vi "Autonomous Independent.vi"() -> ()   [LabVIEW 2014]
doc: "This VI is called when autonomous begins, and will automatically be terminated when autonomous ends. You can carry out timed or sensor driven robot movement independently without needing to return to the caller."
uses:
  <vilib>/Rock Robotics/WPI/Solenoid/WPI_SolenoidValue.ctl
  <vilib>/Rock Robotics/WPI/Solenoid/WPI_SolenoidSetEnum.vi
  <vilib>/Rock Robotics/WPI/RobotDrive/WPI_RobotDriveGetSetRefNum.vi
  <vilib>/Rock Robotics/WPI/RobotDrive/WPI_RobotDriveArcadeDrive_Standard(NoSaturation).vi
panel:
  out "Out":dbl
  # "Be sure to right-click and choose Data Operations>>Make Current Value default if you want to save the array values with the VI"
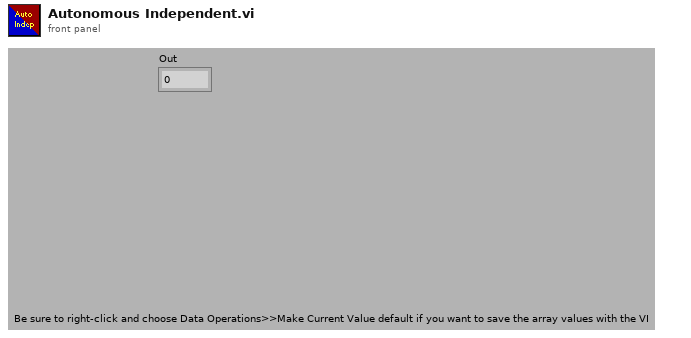
[diagram p1: front panel]
types:
  T1 = typedef "WPI_DigitalInputDevRef.ctl" = cluster{"DevStatus":errorcluster, "DIO Channel":T2, "Controller":T3}
  T2 = typedef "FPGA_DIOChannel.ctl" = enum8{"DIO 0", "DIO 1", "DIO 2", "DIO 3", "DIO 4", "DIO 5", "DIO 6", "DIO 7", "DIO 8", "DIO 9", "DIO MXP 0", "DIO MXP 1", "DIO MXP 2", "DIO MXP 3", "DIO MXP 4", "DIO MXP 5", "DIO MXP 6", "DIO MXP 7", "DIO MXP 8", "DIO MXP 9", "DIO MXP 10", "DIO MXP 11", "DIO MXP 12", "DIO MXP 13", "DIO MXP 14", "DIO MXP 15", "Invalid"}
  T3 = typedef "FPGA_TypedefDigitalModule.ctl" = enum16{"Controller 1"}
  T4 = typedef "WPI_SolenoidValue.ctl" = enum16{"Off", "On", "Forward", "Reverse"}
  T5 = typedef "WPI_SolenoidDevRef.ctl" = cluster{"DevStatus":errorcluster, "Pneumatics Control Module":u8, "Forward Solenoid Channel":T6, "Reverse Solenoid Channel":T6}
  T6 = typedef "WPI_SolenoidChannel.ctl" = enum8{"Solenoid 0", "Solenoid 1", "Solenoid 2", "Solenoid 3", "Solenoid 4", "Solenoid 5", "Solenoid 6", "Solenoid 7", "Invalid"}
  T7 = typedef "WPI_EncoderDevRef.ctl" = cluster{"DevStatus":errorcluster, "EncoderIndex":T8, "CounterIndex":T9, "DistancePerCount":dbl, "Decoding Type":T10}
  T8 = typedef "FPGA_EncoderIdx.ctl" = enum8{"Enc 0", "Enc 1", "Enc 2", "Enc 3", "Enc 4", "Enc 5", "Enc 6", "Enc 7", "Invalid"}
  T9 = typedef "FPGA_CounterCtrSystemIndex.ctl" = enum8{"Ctr 0", "Ctr 1", "Ctr 2", "Ctr 3", "Ctr 4", "Ctr 5", "Ctr 6", "Ctr 7", "Invalid"}
  T10 = typedef "WPI_EncoderType.ctl" = enum16{"1x", "2x", "4x"}
  T11 = typedef "WPI_RobotDriveDevRef.ctl" = cluster{"DevStatus":errorcluster, "Motors[]":T12[], "Square Inputs":bool, "Max Output":dbl}
  T12 = typedef "WPI_MotorControlDeviceRef.ctl" = cluster{"DeviceStatus":errorcluster, "Type":T13, "PWM":cluster{"Controller":T3, "PWM Channel":T14, "DeadBand":T15}, "CAN":cluster{"Device Number":u8, "Control Mode":T16, "Semaphore":T17, "Max Vout":dbl, "TalonSRX Control Mode":T18}, "Invert":bool, "TransformRef":T19, "InvTransformRef":T19}
  T13 = typedef "WPI_MotorControlType.ctl" = enum16{"PWM", "CAN", "CANTalonSRX"}
  T14 = typedef "FPGA_DIOPWMChannel.ctl" = enum8{"PWM 0", "PWM 1", "PWM 2", "PWM 3", "PWM 4", "PWM 5", "PWM 6", "PWM 7", "PWM 8", "PWM 9", "PWM MXP 0", "PWM MXP 1", "PWM MXP 2", "PWM MXP 3", "PWM MXP 4", "PWM MXP 5", "PWM MXP 6", "PWM MXP 7", "PWM MXP 8", "PWM MXP 9", "Invalid"}
  T15 = typedef "WPI_PWMDeadband.ctl" = cluster{"Name":string, "maxPositivePwm":i32, "minPositivePwm":i32, "centerPwm":i32, "maxNegativePwm":i32, "minNegativePwm":i32, "angularRange":u16}
  T16 = typedef "WPI_CANJaguar_ControlMode.ctl" = enum8{"Percent VBus", "Current", "Speed", "Position", "Voltage"}
  T17 = typedef "Semaphore RefNum" = refnum<k1>
  T18 = typedef "WPI_CANTalonSRX_APIControlMode.ctl" = enum8{"Percent VBus", "Speed", "Position", "Slave", "Unchanged / Invalid"}
  T19 = typedef "WPI_PWMTransform_ConPane.ctl" = refnum<vi>
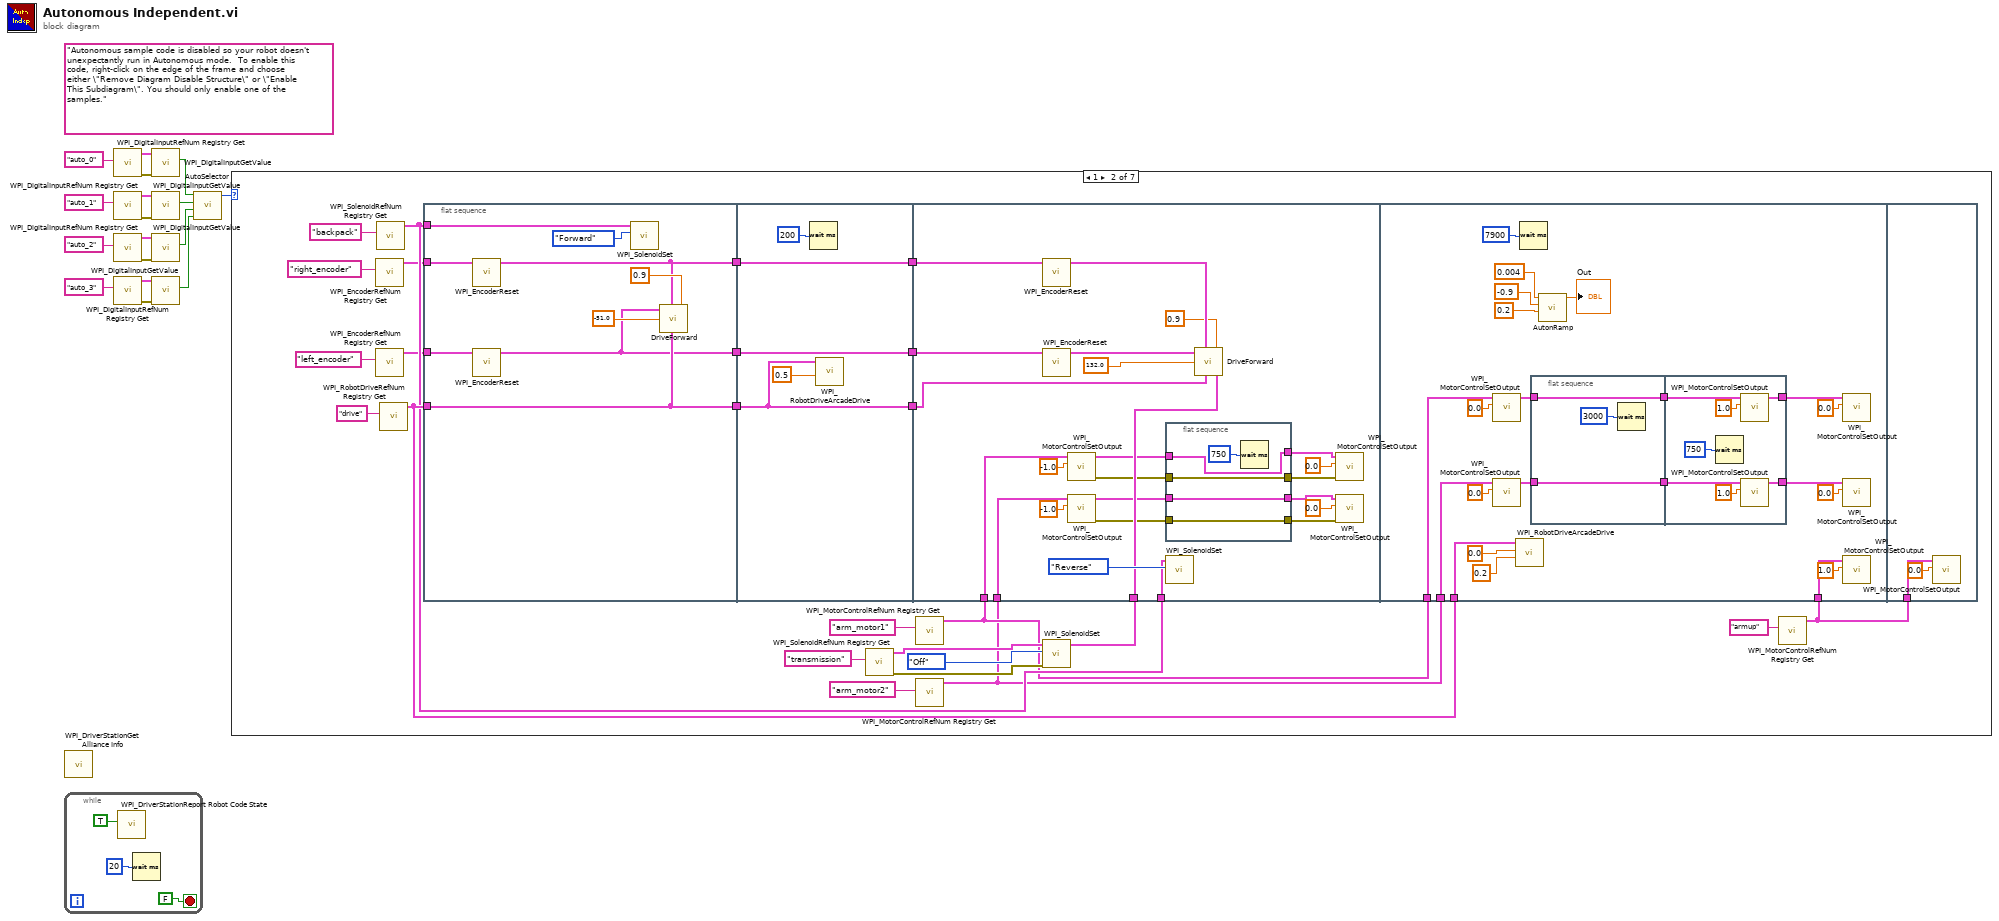
[diagram p0: block diagram]
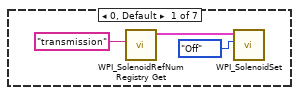
[diagram p2: hidden frame]
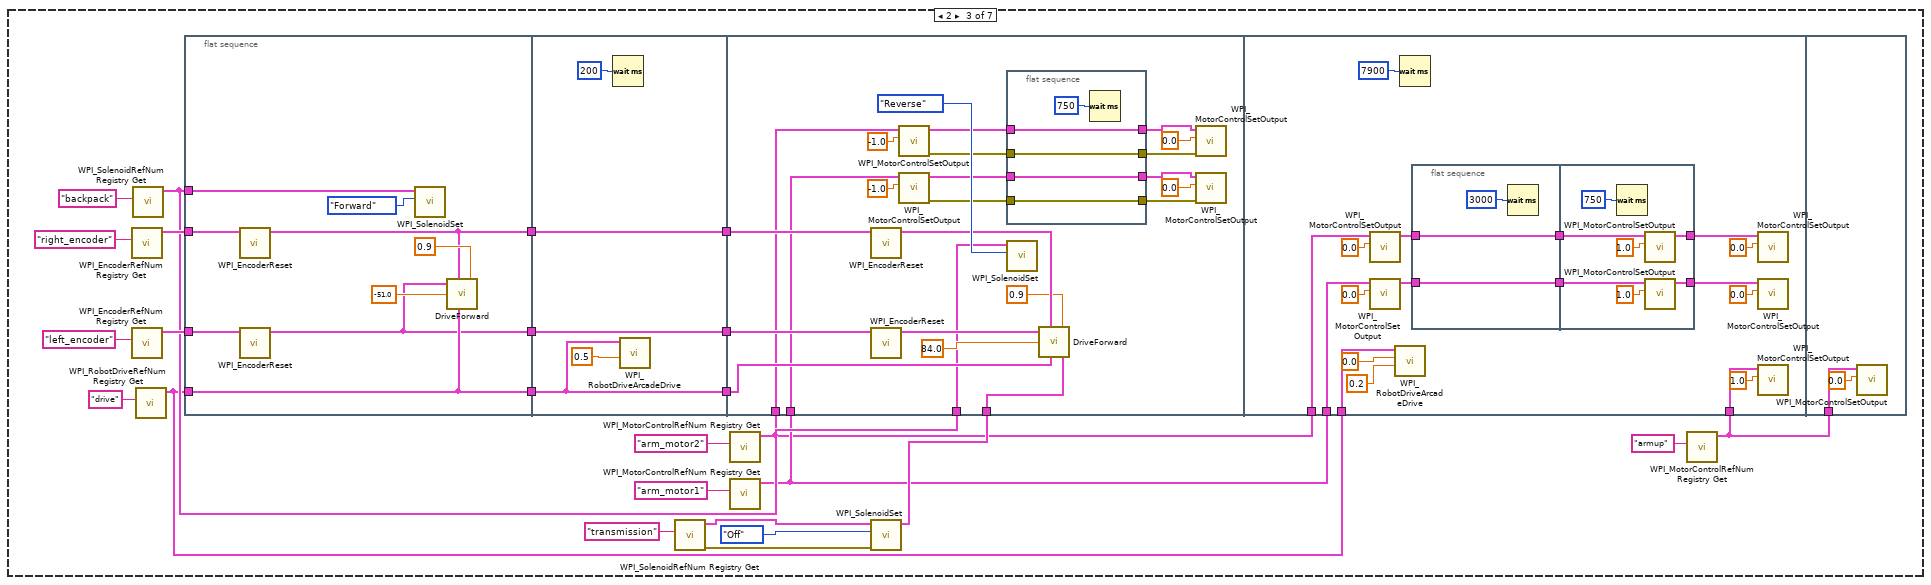
[diagram p3: hidden frame]
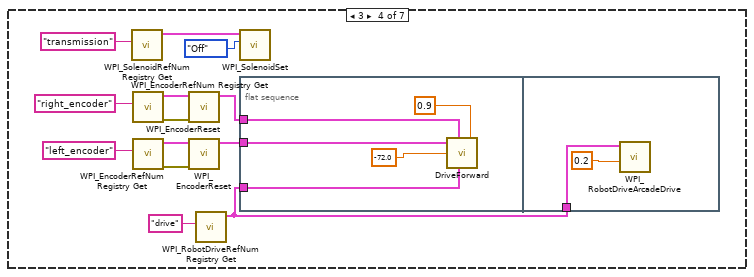
[diagram p4: hidden frame]
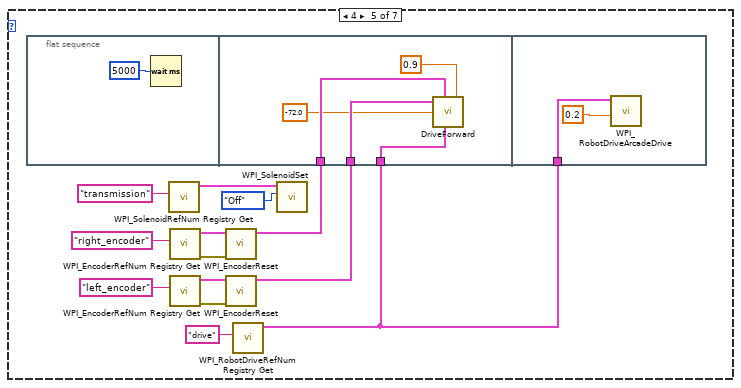
[diagram p5: hidden frame]
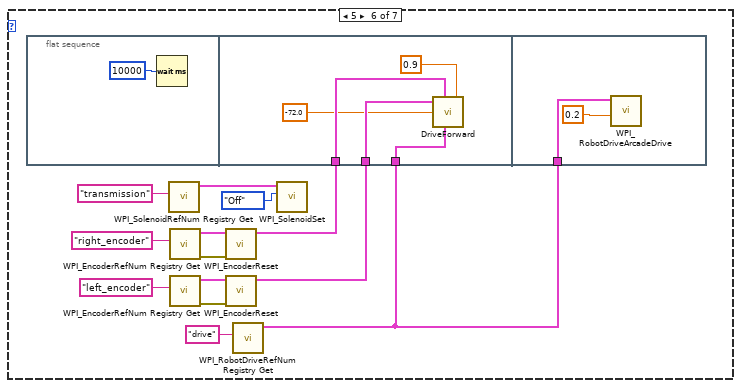
[diagram p6: hidden frame]
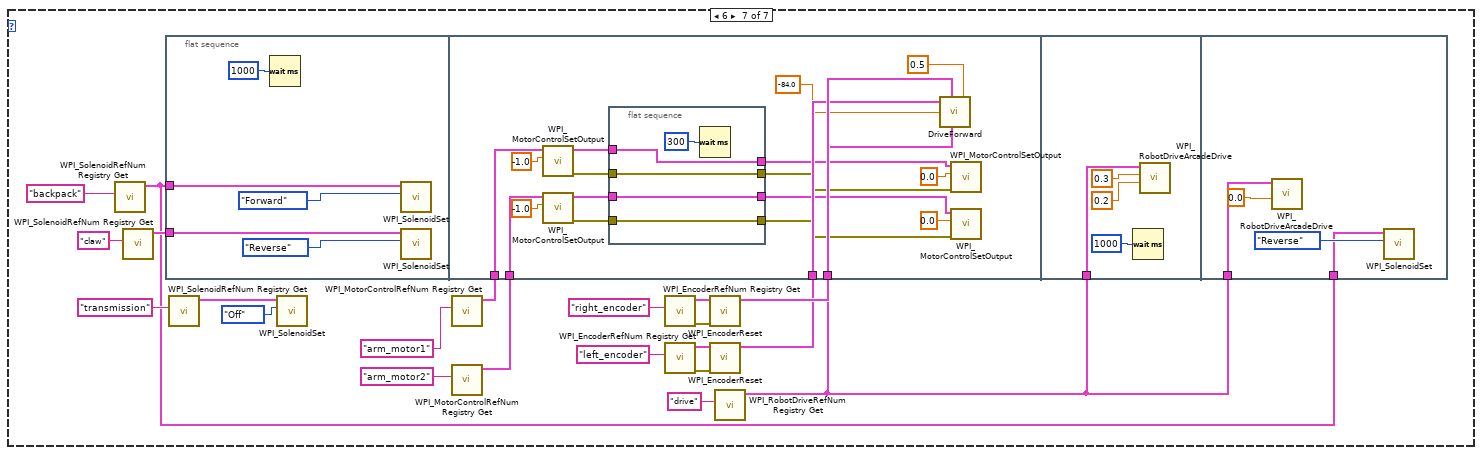
[diagram p7: hidden frame]
diagram:
  (unwired) "Autonomous sample code is disabled so your robot doesn't unexpectantly run in Autonomous mode.  To enable this code, right-click on the edge of the frame and choose either \"Remove Diagram Disable Structure\" or \"Enable This Subdiagram\". You should only enable one of the samples."
  n1 = call <vilib>:"WPI_DriverStationGet Alliance Info.vi"() -> ()  [unwired: 12 out]
  n2 = while {
    stop <- FALSE stop-if-true
    n3 = call <vilib>:"WPI_DriverStationReport Robot Code State.vi"("Autonomous"=TRUE) -> ()  [unwired: 10 in, 1 out]
    n4 = Wait (ms)(milliseconds to wait=u32 20) -> ()  [unwired: 1 out]
  }
  n5 = call <vilib>:"WPI_DigitalInputRefNum Registry Get.vi"("refnum name"="auto_0") -> ("error out"=w16:errorcluster, "DigitalInputDevRef"=w15:T1)  [unwired: 9 in]
  n6 = call <vilib>:"WPI_DigitalInputRefNum Registry Get.vi"("refnum name"="auto_1") -> ("error out"=w13:errorcluster, "DigitalInputDevRef"=w14:T1)  [unwired: 9 in]
  n7 = call <vilib>:"WPI_DigitalInputRefNum Registry Get.vi"("refnum name"="auto_2") -> ("error out"=w11:errorcluster, "DigitalInputDevRef"=w12:T1)  [unwired: 9 in]
  n8 = call <vilib>:"WPI_DigitalInputRefNum Registry Get.vi"("refnum name"="auto_3") -> ("error out"=w9:errorcluster, "DigitalInputDevRef"=w10:T1)  [unwired: 9 in]
  n9 = call <vilib>:"WPI_DigitalInputGetValue.vi"("error in (no error)"=w16, "DigitalInputDevRef"=w15) -> ("Value"=w5:bool)  [unwired: 7 in, 2 out]
  n10 = call <vilib>:"WPI_DigitalInputGetValue.vi"("error in (no error)"=w13, "DigitalInputDevRef"=w14) -> ("Value"=w6:bool)  [unwired: 7 in, 2 out]
  n11 = call <vilib>:"WPI_DigitalInputGetValue.vi"("error in (no error)"=w11, "DigitalInputDevRef"=w12) -> ("Value"=w7:bool)  [unwired: 7 in, 2 out]
  n12 = call <vilib>:"WPI_DigitalInputGetValue.vi"("error in (no error)"=w9, "DigitalInputDevRef"=w10) -> ("Value"=w8:bool)  [unwired: 7 in, 2 out]
  n13 = call "AutoSelector.vi"("3"=w8, "2"=w7, "1"=w6, "0"=w5) -> ("Auto"=w17:i32)  [unwired: 7 in]
  n14 = case shown="1" w17 {
    frame 0, Default {
      n15 = call <vilib>:"WPI_SolenoidRefNum Registry Get.vi"("refnum name"="transmission") -> ("SolenoidDevRef"=w21:T5)  [unwired: 9 in, 1 out]
      n16 = call-poly <vilib>:"WPI_SolenoidSet.vi"("Value"=WPI_SolenoidValue."Off", "SolenoidDevRef"=w21) -> ()  [unwired: 8 in, 2 out]
    }
    frame 1 {
      n17 = call <vilib>:"WPI_EncoderRefNum Registry Get.vi"("refnum name"="right_encoder") -> ("EncoderDevRef"=w34:T7)  [unwired: 9 in, 1 out]
      n18 = call <vilib>:"WPI_EncoderRefNum Registry Get.vi"("refnum name"="left_encoder") -> ("EncoderDevRef"=w35:T7)  [unwired: 9 in, 1 out]
      n19 = call <vilib>:"WPI_SolenoidRefNum Registry Get.vi"("refnum name"="backpack") -> ("SolenoidDevRef"=w36:T5)  [unwired: 9 in, 1 out]
      n20 = call <vilib>:"WPI_RobotDriveRefNum Registry Get.vi"("refnum name"="drive") -> ("RobotDriveDevRef"=w42:T11)  [unwired: 9 in, 1 out]
      n21 = flat-sequence {
        tunnel: w42 -> [w53]
        tunnel: w34 -> [w49]
        tunnel: w35 -> [w50]
        tunnel: w36 -> [w57]
        tunnel: [w53] -> w48
        tunnel: [w52] -> w47
        tunnel: [w51] -> w46
        tunnel: w48 -> [w59]
        tunnel: [w59] -> w45
        tunnel: w47 -> [w62]
        tunnel: [w62] -> w44
        tunnel: w46 -> [w61]
        tunnel: [w61] -> w43
        tunnel: w45 -> [w81]
        tunnel: w44 -> [w80]
        tunnel: w43 -> [w79]
        tunnel: w36 -> [w78]
        tunnel: w37 -> [w77]
        tunnel: w25 -> [w64]
        tunnel: w24 -> [w63]
        tunnel: w41 -> [w111]
        tunnel: w42 -> [w108]
        tunnel: w25 -> [w93]
        tunnel: w24 -> [w92]
        tunnel: w41 -> [w124]
        frame #0 {
          n22 = call <vilib>:"WPI_EncoderReset.vi"("EncoderDevRef"=w49) -> ("EncoderDevRef"=w51:T7)  [unwired: 9 in, 1 out]
          n23 = call <vilib>:"WPI_EncoderReset.vi"("EncoderDevRef"=w50) -> ("EncoderDevRef"=w52:T7)  [unwired: 9 in, 1 out]
          n24 = call-poly <vilib>:"WPI_SolenoidSet.vi"("Value"=WPI_SolenoidValue."Forward", "SolenoidDevRef"=w57) -> ()  [unwired: 8 in, 2 out]
          n25 = call "DriveForward.vi"("LeftEncoder"=w52, "RightEncoder"=w51, "Inches to Travel"=-51.0, "Drive"=w53, "Max"=0.9) -> ()  [unwired: 2 in]
        }
        frame #1 {
          n26 = Wait (ms)(milliseconds to wait=u32 200) -> ()  [unwired: 1 out]
          n27 = call-poly <vilib>:"WPI_RobotDriveArcadeDrive.vi"("Y axis value"=0.5, "RobotDriveDevRef"=w59) -> ()  [unwired: 7 in, 3 out]
        }
        frame #2 {
          n28 = call <vilib>:"WPI_EncoderReset.vi"("EncoderDevRef"=w79) -> ("EncoderDevRef"=w84:T7)  [unwired: 9 in, 1 out]
          n29 = call <vilib>:"WPI_EncoderReset.vi"("EncoderDevRef"=w80) -> ("EncoderDevRef"=w85:T7)  [unwired: 9 in, 1 out]
          n30 = call <vilib>:"WPI_MotorControlSetOutput.vi"("Output"=-1.0, "MotorControlDevRef"=w64) -> ("error out"=w68:errorcluster, "MotorControlDevRef"=w76:T12)  [unwired: 7 in, 1 out]
          n31 = call <vilib>:"WPI_MotorControlSetOutput.vi"("Output"=-1.0, "MotorControlDevRef"=w63) -> ("error out"=w67:errorcluster, "MotorControlDevRef"=w73:T12)  [unwired: 7 in, 1 out]
          n32 = flat-sequence {
            tunnel: w67 -> [w90]
            tunnel: w68 -> [w91]
            tunnel: [w91] -> w69
            tunnel: [w90] -> w70
            tunnel: w73 -> [w88]
            tunnel: [w88] -> w74
            tunnel: [w87] -> w75
            tunnel: w76 -> [w87]
            frame #0 {
              n33 = Wait (ms)(milliseconds to wait=u32 750) -> ()  [unwired: 1 out]
            }
          }
          n34 = call-poly <vilib>:"WPI_SolenoidSet.vi"("Value"=WPI_SolenoidValue."Reverse", "SolenoidDevRef"=w78) -> ()  [unwired: 8 in, 2 out]
          n35 = call "DriveForward.vi"("LeftEncoder"=w85, "RightEncoder"=w84, "Inches to Travel"=132.0, "Drive"=w81, "Max"=0.9, "Transmission"=w77) -> ()  [unwired: 1 in]
          n36 = call <vilib>:"WPI_MotorControlSetOutput.vi"("error in (no error)"=w69, "Output"=0.0, "MotorControlDevRef"=w75) -> ()  [unwired: 6 in, 3 out]
          n37 = call <vilib>:"WPI_MotorControlSetOutput.vi"("error in (no error)"=w70, "Output"=0.0, "MotorControlDevRef"=w74) -> ()  [unwired: 6 in, 3 out]
        }
        frame #3 {
          n38 = call <vilib>:"WPI_MotorControlSetOutput.vi"("Output"=0.0, "MotorControlDevRef"=w93) -> ("MotorControlDevRef"=w98:T12)  [unwired: 7 in, 2 out]
          n39 = call <vilib>:"WPI_MotorControlSetOutput.vi"("Output"=0.0, "MotorControlDevRef"=w92) -> ("MotorControlDevRef"=w99:T12)  [unwired: 7 in, 2 out]
          n40 = call-poly <vilib>:"WPI_RobotDriveArcadeDrive.vi"("Y axis value"=0.2, "X axis value"=0.0 ("Y axis value"), "RobotDriveDevRef"=w108) -> ()  [unwired: 6 in, 3 out]
          n41 = Wait (ms)(milliseconds to wait=u32 7900) -> ()  [unwired: 1 out]
          n42 = flat-sequence {
            tunnel: w99 -> [w115]
            tunnel: w98 -> [w114]
            tunnel: [w115] -> w103
            tunnel: [w114] -> w102
            tunnel: w103 -> [w120]
            tunnel: w102 -> [w119]
            tunnel: [w117] -> w96
            tunnel: [w118] -> w97
            frame #0 {
              n43 = Wait (ms)(milliseconds to wait=u32 3000) -> ()  [unwired: 1 out]
            }
            frame #1 {
              n44 = Wait (ms)(milliseconds to wait=u32 750) -> ()  [unwired: 1 out]
              n45 = call <vilib>:"WPI_MotorControlSetOutput.vi"("Output"=1.0, "MotorControlDevRef"=w119) -> ("MotorControlDevRef"=w117:T12)  [unwired: 7 in, 2 out]
              n46 = call <vilib>:"WPI_MotorControlSetOutput.vi"("Output"=1.0, "MotorControlDevRef"=w120) -> ("MotorControlDevRef"=w118:T12)  [unwired: 7 in, 2 out]
            }
          }
          n47 = call "AutonRamp.vi"("Target"=0.2, "Start"=-0.9, "Rate"=0.004) -> ("Out"=→"Out":dbl)  [unwired: 8 in]
          n48 = call <vilib>:"WPI_MotorControlSetOutput.vi"("Output"=0.0, "MotorControlDevRef"=w96) -> ()  [unwired: 7 in, 3 out]
          n49 = call <vilib>:"WPI_MotorControlSetOutput.vi"("Output"=0.0, "MotorControlDevRef"=w97) -> ()  [unwired: 7 in, 3 out]
          n50 = call <vilib>:"WPI_MotorControlSetOutput.vi"("Output"=1.0, "MotorControlDevRef"=w111) -> ()  [unwired: 7 in, 3 out]
        }
        frame #4 {
          n51 = call <vilib>:"WPI_MotorControlSetOutput.vi"("Output"=0.0, "MotorControlDevRef"=w124) -> ()  [unwired: 7 in, 3 out]
        }
      }
      n52 = call <vilib>:"WPI_SolenoidRefNum Registry Get.vi"("refnum name"="transmission") -> ("error out"=w29:errorcluster, "SolenoidDevRef"=w30:T5)  [unwired: 9 in]
      n53 = call <vilib>:"WPI_MotorControlRefNum Registry Get.vi"("refnum name"="arm_motor1") -> ("MotorControlDevRef"=w25:T12)  [unwired: 9 in, 1 out]
      n54 = call <vilib>:"WPI_MotorControlRefNum Registry Get.vi"("refnum name"="arm_motor2") -> ("MotorControlDevRef"=w24:T12)  [unwired: 9 in, 1 out]
      n55 = call-poly <vilib>:"WPI_SolenoidSet.vi"("error in (no error)"=w29, "Value"=WPI_SolenoidValue."Off", "SolenoidDevRef"=w30) -> ("SolenoidDevRef"=w37:T5)  [unwired: 7 in, 1 out]
      n56 = call <vilib>:"WPI_MotorControlRefNum Registry Get.vi"("refnum name"="armup") -> ("MotorControlDevRef"=w41:T12)  [unwired: 9 in, 1 out]
    }
    frame 2 {
      n57 = call <vilib>:"WPI_EncoderRefNum Registry Get.vi"("refnum name"="right_encoder") -> ("EncoderDevRef"=w136:T7)  [unwired: 9 in, 1 out]
      n58 = call <vilib>:"WPI_EncoderRefNum Registry Get.vi"("refnum name"="left_encoder") -> ("EncoderDevRef"=w135:T7)  [unwired: 9 in, 1 out]
      n59 = call <vilib>:"WPI_SolenoidRefNum Registry Get.vi"("refnum name"="backpack") -> ("SolenoidDevRef"=w134:T5)  [unwired: 9 in, 1 out]
      n60 = call <vilib>:"WPI_RobotDriveRefNum Registry Get.vi"("refnum name"="drive") -> ("RobotDriveDevRef"=w128:T11)  [unwired: 9 in, 1 out]
      n61 = flat-sequence {
        tunnel: w128 -> [w155]
        tunnel: w136 -> [w151]
        tunnel: w135 -> [w152]
        tunnel: w134 -> [w159]
        tunnel: [w155] -> w150
        tunnel: [w154] -> w149
        tunnel: [w153] -> w148
        tunnel: w150 -> [w161]
        tunnel: [w161] -> w147
        tunnel: w149 -> [w164]
        tunnel: [w164] -> w146
        tunnel: w148 -> [w163]
        tunnel: [w163] -> w145
        tunnel: w147 -> [w183]
        tunnel: w146 -> [w182]
        tunnel: w145 -> [w181]
        tunnel: w134 -> [w180]
        tunnel: w133 -> [w179]
        tunnel: w127 -> [w166]
        tunnel: w126 -> [w165]
        tunnel: w129 -> [w209]
        tunnel: w128 -> [w206]
        tunnel: w127 -> [w203]
        tunnel: w126 -> [w202]
        tunnel: w129 -> [w222]
        frame #0 {
          n62 = call <vilib>:"WPI_EncoderReset.vi"("EncoderDevRef"=w151) -> ("EncoderDevRef"=w153:T7)  [unwired: 9 in, 1 out]
          n63 = call <vilib>:"WPI_EncoderReset.vi"("EncoderDevRef"=w152) -> ("EncoderDevRef"=w154:T7)  [unwired: 9 in, 1 out]
          n64 = call-poly <vilib>:"WPI_SolenoidSet.vi"("Value"=WPI_SolenoidValue."Forward", "SolenoidDevRef"=w159) -> ()  [unwired: 8 in, 2 out]
          n65 = call "DriveForward.vi"("LeftEncoder"=w154, "RightEncoder"=w153, "Inches to Travel"=-51.0, "Drive"=w155, "Max"=0.9) -> ()  [unwired: 2 in]
        }
        frame #1 {
          n66 = Wait (ms)(milliseconds to wait=u32 200) -> ()  [unwired: 1 out]
          n67 = call-poly <vilib>:"WPI_RobotDriveArcadeDrive.vi"("Y axis value"=0.5, "RobotDriveDevRef"=w161) -> ()  [unwired: 7 in, 3 out]
        }
        frame #2 {
          n68 = call <vilib>:"WPI_EncoderReset.vi"("EncoderDevRef"=w181) -> ("EncoderDevRef"=w186:T7)  [unwired: 9 in, 1 out]
          n69 = call <vilib>:"WPI_EncoderReset.vi"("EncoderDevRef"=w182) -> ("EncoderDevRef"=w187:T7)  [unwired: 9 in, 1 out]
          n70 = call <vilib>:"WPI_MotorControlSetOutput.vi"("Output"=-1.0, "MotorControlDevRef"=w165) -> ("error out"=w169:errorcluster, "MotorControlDevRef"=w175:T12)  [unwired: 7 in, 1 out]
          n71 = call <vilib>:"WPI_MotorControlSetOutput.vi"("Output"=-1.0, "MotorControlDevRef"=w166) -> ("error out"=w170:errorcluster, "MotorControlDevRef"=w178:T12)  [unwired: 7 in, 1 out]
          n72 = flat-sequence {
            tunnel: w169 -> [w192]
            tunnel: w170 -> [w193]
            tunnel: [w193] -> w171
            tunnel: [w192] -> w172
            tunnel: w175 -> [w190]
            tunnel: [w190] -> w176
            tunnel: [w189] -> w177
            tunnel: w178 -> [w189]
            frame #0 {
              n73 = Wait (ms)(milliseconds to wait=u32 750) -> ()  [unwired: 1 out]
            }
          }
          n74 = call-poly <vilib>:"WPI_SolenoidSet.vi"("Value"=WPI_SolenoidValue."Reverse", "SolenoidDevRef"=w180) -> ()  [unwired: 8 in, 2 out]
          n75 = call "DriveForward.vi"("LeftEncoder"=w187, "RightEncoder"=w186, "Inches to Travel"=84.0, "Drive"=w183, "Max"=0.9, "Transmission"=w179) -> ()  [unwired: 1 in]
          n76 = call <vilib>:"WPI_MotorControlSetOutput.vi"("error in (no error)"=w172, "Output"=0.0, "MotorControlDevRef"=w176) -> ()  [unwired: 6 in, 3 out]
          n77 = call <vilib>:"WPI_MotorControlSetOutput.vi"("error in (no error)"=w171, "Output"=0.0, "MotorControlDevRef"=w177) -> ()  [unwired: 6 in, 3 out]
        }
        frame #3 {
          n78 = call <vilib>:"WPI_MotorControlSetOutput.vi"("Output"=0.0, "MotorControlDevRef"=w202) -> ("MotorControlDevRef"=w200:T12)  [unwired: 7 in, 2 out]
          n79 = call <vilib>:"WPI_MotorControlSetOutput.vi"("Output"=0.0, "MotorControlDevRef"=w203) -> ("MotorControlDevRef"=w201:T12)  [unwired: 7 in, 2 out]
          n80 = call-poly <vilib>:"WPI_RobotDriveArcadeDrive.vi"("Y axis value"=0.2, "X axis value"=0.0 ("Y axis value"), "RobotDriveDevRef"=w206) -> ()  [unwired: 6 in, 3 out]
          n81 = Wait (ms)(milliseconds to wait=u32 7900) -> ()  [unwired: 1 out]
          n82 = flat-sequence {
            tunnel: w201 -> [w213]
            tunnel: w200 -> [w212]
            tunnel: [w213] -> w199
            tunnel: [w212] -> w198
            tunnel: w199 -> [w218]
            tunnel: w198 -> [w217]
            tunnel: [w215] -> w196
            tunnel: [w216] -> w197
            frame #0 {
              n83 = Wait (ms)(milliseconds to wait=u32 3000) -> ()  [unwired: 1 out]
            }
            frame #1 {
              n84 = Wait (ms)(milliseconds to wait=u32 750) -> ()  [unwired: 1 out]
              n85 = call <vilib>:"WPI_MotorControlSetOutput.vi"("Output"=1.0, "MotorControlDevRef"=w217) -> ("MotorControlDevRef"=w215:T12)  [unwired: 7 in, 2 out]
              n86 = call <vilib>:"WPI_MotorControlSetOutput.vi"("Output"=1.0, "MotorControlDevRef"=w218) -> ("MotorControlDevRef"=w216:T12)  [unwired: 7 in, 2 out]
            }
          }
          n87 = call <vilib>:"WPI_MotorControlSetOutput.vi"("Output"=0.0, "MotorControlDevRef"=w196) -> ()  [unwired: 7 in, 3 out]
          n88 = call <vilib>:"WPI_MotorControlSetOutput.vi"("Output"=0.0, "MotorControlDevRef"=w197) -> ()  [unwired: 7 in, 3 out]
          n89 = call <vilib>:"WPI_MotorControlSetOutput.vi"("Output"=1.0, "MotorControlDevRef"=w209) -> ()  [unwired: 7 in, 3 out]
        }
        frame #4 {
          n90 = call <vilib>:"WPI_MotorControlSetOutput.vi"("Output"=0.0, "MotorControlDevRef"=w222) -> ()  [unwired: 7 in, 3 out]
        }
      }
      n91 = call <vilib>:"WPI_SolenoidRefNum Registry Get.vi"("refnum name"="transmission") -> ("error out"=w141:errorcluster, "SolenoidDevRef"=w140:T5)  [unwired: 9 in]
      n92 = call <vilib>:"WPI_MotorControlRefNum Registry Get.vi"("refnum name"="arm_motor2") -> ("MotorControlDevRef"=w126:T12)  [unwired: 9 in, 1 out]
      n93 = call <vilib>:"WPI_MotorControlRefNum Registry Get.vi"("refnum name"="arm_motor1") -> ("MotorControlDevRef"=w127:T12)  [unwired: 9 in, 1 out]
      n94 = call-poly <vilib>:"WPI_SolenoidSet.vi"("error in (no error)"=w141, "Value"=WPI_SolenoidValue."Off", "SolenoidDevRef"=w140) -> ("SolenoidDevRef"=w133:T5)  [unwired: 7 in, 1 out]
      n95 = call <vilib>:"WPI_MotorControlRefNum Registry Get.vi"("refnum name"="armup") -> ("MotorControlDevRef"=w129:T12)  [unwired: 9 in, 1 out]
    }
    frame 3 {
      n96 = call <vilib>:"WPI_SolenoidRefNum Registry Get.vi"("refnum name"="transmission") -> ("SolenoidDevRef"=w224:T5)  [unwired: 9 in, 1 out]
      n97 = call <vilib>:"WPI_EncoderRefNum Registry Get.vi"("refnum name"="right_encoder") -> ("error out"=w229:errorcluster, "EncoderDevRef"=w232:T7)  [unwired: 9 in]
      n98 = call <vilib>:"WPI_EncoderRefNum Registry Get.vi"("refnum name"="left_encoder") -> ("error out"=w230:errorcluster, "EncoderDevRef"=w231:T7)  [unwired: 9 in]
      n99 = call <vilib>:"WPI_EncoderReset.vi"("error in (no error)"=w229, "EncoderDevRef"=w232) -> ("EncoderDevRef"=w228:T7)  [unwired: 8 in, 1 out]
      n100 = call <vilib>:"WPI_EncoderReset.vi"("error in (no error)"=w230, "EncoderDevRef"=w231) -> ("EncoderDevRef"=w227:T7)  [unwired: 8 in, 1 out]
      n101 = call <vilib>:"WPI_RobotDriveRefNum Registry Get.vi"("refnum name"="drive") -> ("RobotDriveDevRef"=w235:T11)  [unwired: 9 in, 1 out]
      n102 = call-poly <vilib>:"WPI_SolenoidSet.vi"("Value"=WPI_SolenoidValue."Off", "SolenoidDevRef"=w224) -> ()  [unwired: 8 in, 2 out]
      n103 = flat-sequence {
        tunnel: w235 -> [w238]
        tunnel: w228 -> [w241]
        tunnel: w227 -> [w240]
        tunnel: w235 -> [w243]
        frame #0 {
          n104 = call "DriveForward.vi"("LeftEncoder"=w240, "RightEncoder"=w241, "Inches to Travel"=-72.0, "Drive"=w238, "Max"=0.9) -> ()  [unwired: 2 in]
        }
        frame #1 {
          n105 = call-poly <vilib>:"WPI_RobotDriveArcadeDrive.vi"("Y axis value"=0.2, "RobotDriveDevRef"=w243) -> ()  [unwired: 7 in, 3 out]
        }
      }
    }
    frame 4 {
      n106 = flat-sequence {
        tunnel: w255 -> [w259]
        tunnel: w248 -> [w262]
        tunnel: w247 -> [w261]
        tunnel: w255 -> [w264]
        frame #0 {
          n107 = Wait (ms)(milliseconds to wait=u32 5000) -> ()  [unwired: 1 out]
        }
        frame #1 {
          n108 = call "DriveForward.vi"("LeftEncoder"=w261, "RightEncoder"=w262, "Inches to Travel"=-72.0, "Drive"=w259, "Max"=0.9) -> ()  [unwired: 2 in]
        }
        frame #2 {
          n109 = call-poly <vilib>:"WPI_RobotDriveArcadeDrive.vi"("Y axis value"=0.2, "RobotDriveDevRef"=w264) -> ()  [unwired: 7 in, 3 out]
        }
      }
      n110 = call <vilib>:"WPI_SolenoidRefNum Registry Get.vi"("refnum name"="transmission") -> ("SolenoidDevRef"=w244:T5)  [unwired: 9 in, 1 out]
      n111 = call <vilib>:"WPI_EncoderRefNum Registry Get.vi"("refnum name"="right_encoder") -> ("error out"=w249:errorcluster, "EncoderDevRef"=w252:T7)  [unwired: 9 in]
      n112 = call <vilib>:"WPI_EncoderRefNum Registry Get.vi"("refnum name"="left_encoder") -> ("error out"=w250:errorcluster, "EncoderDevRef"=w251:T7)  [unwired: 9 in]
      n113 = call <vilib>:"WPI_EncoderReset.vi"("error in (no error)"=w249, "EncoderDevRef"=w252) -> ("EncoderDevRef"=w248:T7)  [unwired: 8 in, 1 out]
      n114 = call <vilib>:"WPI_EncoderReset.vi"("error in (no error)"=w250, "EncoderDevRef"=w251) -> ("EncoderDevRef"=w247:T7)  [unwired: 8 in, 1 out]
      n115 = call <vilib>:"WPI_RobotDriveRefNum Registry Get.vi"("refnum name"="drive") -> ("RobotDriveDevRef"=w255:T11)  [unwired: 9 in, 1 out]
      n116 = call-poly <vilib>:"WPI_SolenoidSet.vi"("Value"=WPI_SolenoidValue."Off", "SolenoidDevRef"=w244) -> ()  [unwired: 8 in, 2 out]
    }
    frame 5 {
      n117 = flat-sequence {
        tunnel: w276 -> [w280]
        tunnel: w269 -> [w283]
        tunnel: w268 -> [w282]
        tunnel: w276 -> [w285]
        frame #0 {
          n118 = Wait (ms)(milliseconds to wait=u32 10000) -> ()  [unwired: 1 out]
        }
        frame #1 {
          n119 = call "DriveForward.vi"("LeftEncoder"=w282, "RightEncoder"=w283, "Inches to Travel"=-72.0, "Drive"=w280, "Max"=0.9) -> ()  [unwired: 2 in]
        }
        frame #2 {
          n120 = call-poly <vilib>:"WPI_RobotDriveArcadeDrive.vi"("Y axis value"=0.2, "RobotDriveDevRef"=w285) -> ()  [unwired: 7 in, 3 out]
        }
      }
      n121 = call <vilib>:"WPI_SolenoidRefNum Registry Get.vi"("refnum name"="transmission") -> ("SolenoidDevRef"=w265:T5)  [unwired: 9 in, 1 out]
      n122 = call <vilib>:"WPI_EncoderRefNum Registry Get.vi"("refnum name"="right_encoder") -> ("error out"=w270:errorcluster, "EncoderDevRef"=w273:T7)  [unwired: 9 in]
      n123 = call <vilib>:"WPI_EncoderRefNum Registry Get.vi"("refnum name"="left_encoder") -> ("error out"=w271:errorcluster, "EncoderDevRef"=w272:T7)  [unwired: 9 in]
      n124 = call <vilib>:"WPI_EncoderReset.vi"("error in (no error)"=w270, "EncoderDevRef"=w273) -> ("EncoderDevRef"=w269:T7)  [unwired: 8 in, 1 out]
      n125 = call <vilib>:"WPI_EncoderReset.vi"("error in (no error)"=w271, "EncoderDevRef"=w272) -> ("EncoderDevRef"=w268:T7)  [unwired: 8 in, 1 out]
      n126 = call <vilib>:"WPI_RobotDriveRefNum Registry Get.vi"("refnum name"="drive") -> ("RobotDriveDevRef"=w276:T11)  [unwired: 9 in, 1 out]
      n127 = call-poly <vilib>:"WPI_SolenoidSet.vi"("Value"=WPI_SolenoidValue."Off", "SolenoidDevRef"=w265) -> ()  [unwired: 8 in, 2 out]
    }
    frame 6 {
      n128 = call <vilib>:"WPI_SolenoidRefNum Registry Get.vi"("refnum name"="backpack") -> ("SolenoidDevRef"=w286:T5)  [unwired: 9 in, 1 out]
      n129 = call <vilib>:"WPI_SolenoidRefNum Registry Get.vi"("refnum name"="claw") -> ("SolenoidDevRef"=w293:T5)  [unwired: 9 in, 1 out]
      n130 = flat-sequence {
        tunnel: w293 -> [w311]
        tunnel: w286 -> [w307]
        tunnel: w288 -> [w327]
        tunnel: w299 -> [w330]
        tunnel: w298 -> [w329]
        tunnel: w292 -> [w313]
        tunnel: w291 -> [w312]
        tunnel: w288 -> [w339]
        tunnel: w288 -> [w342]
        tunnel: w286 -> [w340]
        frame #0 {
          n131 = Wait (ms)(milliseconds to wait=u32 1000) -> ()  [unwired: 1 out]
          n132 = call-poly <vilib>:"WPI_SolenoidSet.vi"("Value"=WPI_SolenoidValue."Forward", "SolenoidDevRef"=w307) -> ()  [unwired: 8 in, 2 out]
          n133 = call-poly <vilib>:"WPI_SolenoidSet.vi"("Value"=WPI_SolenoidValue."Reverse", "SolenoidDevRef"=w311) -> ()  [unwired: 8 in, 2 out]
        }
        frame #1 {
          n134 = call <vilib>:"WPI_MotorControlSetOutput.vi"("Output"=-1.0, "MotorControlDevRef"=w313) -> ("error out"=w316:errorcluster, "MotorControlDevRef"=w322:T12)  [unwired: 7 in, 1 out]
          n135 = call <vilib>:"WPI_MotorControlSetOutput.vi"("Output"=-1.0, "MotorControlDevRef"=w312) -> ("error out"=w317:errorcluster, "MotorControlDevRef"=w325:T12)  [unwired: 7 in, 1 out]
          n136 = flat-sequence {
            tunnel: w316 -> [w334]
            tunnel: w317 -> [w335]
            tunnel: [w335] -> w318
            tunnel: [w334] -> w319
            tunnel: w322 -> [w332]
            tunnel: [w332] -> w323
            tunnel: [w331] -> w324
            tunnel: w325 -> [w331]
            frame #0 {
              n137 = Wait (ms)(milliseconds to wait=u32 300) -> ()  [unwired: 1 out]
            }
          }
          n138 = call "DriveForward.vi"("LeftEncoder"=w329, "RightEncoder"=w330, "Inches to Travel"=-84.0, "Drive"=w327, "Max"=0.5) -> ()  [unwired: 2 in]
          n139 = call <vilib>:"WPI_MotorControlSetOutput.vi"("error in (no error)"=w319, "Output"=0.0, "MotorControlDevRef"=w323) -> ()  [unwired: 6 in, 3 out]
          n140 = call <vilib>:"WPI_MotorControlSetOutput.vi"("error in (no error)"=w318, "Output"=0.0, "MotorControlDevRef"=w324) -> ()  [unwired: 6 in, 3 out]
        }
        frame #2 {
          n141 = Wait (ms)(milliseconds to wait=u32 1000) -> ()  [unwired: 1 out]
          n142 = call-poly <vilib>:"WPI_RobotDriveArcadeDrive.vi"("Y axis value"=0.2, "X axis value"=0.3, "RobotDriveDevRef"=w339) -> ()  [unwired: 6 in, 3 out]
        }
        frame #3 {
          n143 = call-poly <vilib>:"WPI_RobotDriveArcadeDrive.vi"("Y axis value"=0.0, "RobotDriveDevRef"=w342) -> ()  [unwired: 7 in, 3 out]
          n144 = call-poly <vilib>:"WPI_SolenoidSet.vi"("Value"=WPI_SolenoidValue."Reverse", "SolenoidDevRef"=w340) -> ()  [unwired: 8 in, 2 out]
        }
      }
      n145 = call <vilib>:"WPI_SolenoidRefNum Registry Get.vi"("refnum name"="transmission") -> ("SolenoidDevRef"=w295:T5)  [unwired: 9 in, 1 out]
      n146 = call-poly <vilib>:"WPI_SolenoidSet.vi"("Value"=WPI_SolenoidValue."Off", "SolenoidDevRef"=w295) -> ()  [unwired: 8 in, 2 out]
      n147 = call <vilib>:"WPI_MotorControlRefNum Registry Get.vi"("refnum name"="arm_motor1") -> ("MotorControlDevRef"=w292:T12)  [unwired: 9 in, 1 out]
      n148 = call <vilib>:"WPI_MotorControlRefNum Registry Get.vi"("refnum name"="arm_motor2") -> ("MotorControlDevRef"=w291:T12)  [unwired: 9 in, 1 out]
      n149 = call <vilib>:"WPI_EncoderRefNum Registry Get.vi"("refnum name"="right_encoder") -> ("error out"=w300:errorcluster, "EncoderDevRef"=w303:T7)  [unwired: 9 in]
      n150 = call <vilib>:"WPI_EncoderRefNum Registry Get.vi"("refnum name"="left_encoder") -> ("error out"=w301:errorcluster, "EncoderDevRef"=w302:T7)  [unwired: 9 in]
      n151 = call <vilib>:"WPI_EncoderReset.vi"("error in (no error)"=w300, "EncoderDevRef"=w303) -> ("EncoderDevRef"=w299:T7)  [unwired: 8 in, 1 out]
      n152 = call <vilib>:"WPI_EncoderReset.vi"("error in (no error)"=w301, "EncoderDevRef"=w302) -> ("EncoderDevRef"=w298:T7)  [unwired: 8 in, 1 out]
      n153 = call <vilib>:"WPI_RobotDriveRefNum Registry Get.vi"("refnum name"="drive") -> ("RobotDriveDevRef"=w288:T11)  [unwired: 9 in, 1 out]
    }
  }
